vi "log-errors.vi"(8 "error in (no error)":errorcluster, 10 "device":string, 11 "refnum in":refnum<file>) -> (0 "error out":errorcluster, 3 "refnum out":refnum<file>)   [LabVIEW 2016]
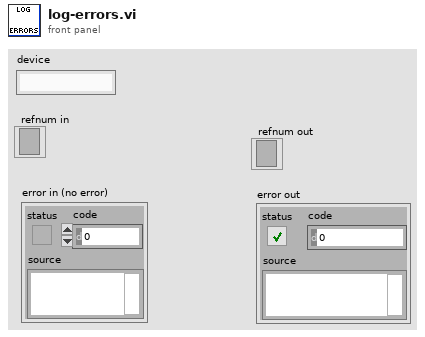
[diagram p1: front panel]
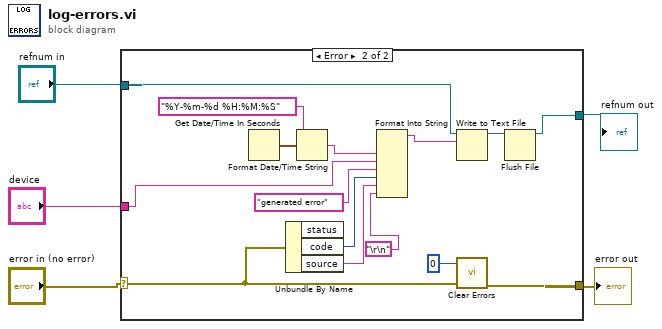
[diagram p0: block diagram]
diagram:
  n1 = case shown="Error" "error in (no error)" {
    selector: "error in (no error)" -> [w6 w20]
    tunnel: [w7 w12] -> w5
    tunnel: "refnum in" -> [w7 w21]
    tunnel: [w6 w19] -> w2
    tunnel: "device" -> [_ w17]
    frame No Error {
    }
    frame Error {
      n2 = Get Date/Time In Seconds() -> (seconds since 1Jan1904=w15:timestamp)
      n3 = Unbundle By Name(w20) -> ("code"=w10:i32, "source"=w9:string)  [unwired: 1 out]
      n4 = Format Date/Time String(time format string (%c)="%Y-%m-%d %H:%M:%S", seconds (now)=w15) -> (date/time string=w16:string)  [unwired: 1 in]
      n5 = Format Into String(w16, w17, "generated error", w10, w9, "\r\n") -> (resulting string=w18:string)  [unwired: 3 in, 1 out]
      n6 = Write to Text File(file (use dialog)=w21, text=w18) -> (refnum out=w13:refnum<file>)  [unwired: 2 in, 2 out]
      n7 = call <vilib>:"Clear Errors.vi"("error in (no error)"=w20, "specific error code to clear (0: all)"=0) -> ("error out"=w19:errorcluster)  [unwired: 4 in, 1 out]
      n8 = Flush File(refnum=w13) -> (refnum out=w12:refnum<file>)  [unwired: 1 in, 1 out]
    }
  }
  "error out" <- w2
  "refnum out" <- w5
